vi "Shooter Code.vi"(10 "velocity_lower":dbl=1.0 format="%#_13g", 11 "velocity_upper":dbl=0.9 format="%#_13g") -> (1 "lowerRPM":dbl, 3 "upperRPM":dbl)   [LabVIEW 2015]
panel:
  in  "index":dbl=1.0
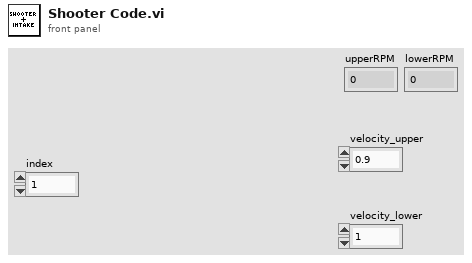
[diagram p1: front panel]
types:
  T1 = typedef "WPI_MotorControlDeviceRef.ctl" = cluster{"DeviceStatus":errorcluster, "Type":T2, "PWM":cluster{"PWM Channel":T3, "DeadBand":T4}, "CAN":cluster{"Device Number":u8, "Control Mode":T5, "Semaphore":T6, "Max Vout":dbl, "TalonSRX Control Mode":T7}, "Invert":bool}
  T2 = typedef "WPI_MotorControlType.ctl" = enum16{"PWM", "CAN", "CANTalonSRX"}
  T3 = typedef "FPGA_DIOPWMChannel.ctl" = enum8{"PWM 0", "PWM 1", "PWM 2", "PWM 3", "PWM 4", "PWM 5", "PWM 6", "PWM 7", "PWM 8", "PWM 9", "PWM MXP 0", "PWM MXP 1", "PWM MXP 2", "PWM MXP 3", "PWM MXP 4", "PWM MXP 5", "PWM MXP 6", "PWM MXP 7", "PWM MXP 8", "PWM MXP 9", "Invalid"}
  T4 = typedef "WPI_PWMDeadband.ctl" = cluster{"Name":string, "maxPositivePwm":i32, "minPositivePwm":i32, "centerPwm":i32, "maxNegativePwm":i32, "minNegativePwm":i32, "angularRange":u16}
  T5 = typedef "WPI_CANJaguar_ControlMode.ctl" = enum8{"Percent VBus", "Current", "Speed", "Position", "Voltage"}
  T6 = typedef "Semaphore RefNum" = refnum<k1>
  T7 = typedef "WPI_CANTalonSRX_APIControlMode.ctl" = enum8{"Percent VBus", "Speed", "Position", "Slave", "Unchanged / Invalid", "Voltage Compensation", "Current", "Motion Profile"}
  T8 = typedef "WPI_CANTalonSRX_GlobalStatus.ctl" = cluster{"Applied Throttle":dbl, "Module Enabled":bool, "CAN Error":errorcluster, "Closed Loop Error":dbl, "Forward Limit Switch Closed":bool, "Reverse Limit Switch Closed":bool, "Sensor Position":dbl, "Sensor Velocity":dbl, "Current":dbl, "Sticky Fault - Over Temp":bool, "Sticky Fault - Under Voltage":bool, "Sticky Fault - Forward Limit":bool, "Sticky Fault - Reverse Limit":bool, "Sticky Fault - Forward Soft Limit":bool, "Sticky Fault - Reverse Soft Limit":bool, "Brake is Enabled":bool, "Encoder Position":dbl, "Encoder Velocity":dbl, "Encoder Index Count":dbl, "Encoder A Pin State":bool, "Encoder B Pin State":bool, "Encoder Index Pin State":bool, "Analog In":dbl, "Analog In Velocity":dbl, "Temperature (C)":dbl, "Battery Voltage":dbl, "Control 5 Is Supported":bool, "Current Profile Slot Select":dbl, "Pos Div 8":bool, "Vel Div 4":bool, "Pulse Width Position":i32, "Pulse Width Velocity":i32, "Pulse Width Rise To Rise (us)":i32, "Pulse Width Rise To Fall (us)":i32, "Mot Prof Active Is Under Run":bool, "Mot Prof Active Has Under Run":bool, "Mot Prof Active Is Last":bool, "Mot Prof Active Velocity Only":bool, "Mot Prof Active Is Valid":bool, "Mot Prof Buffer Is Full":bool, "Mot Prof Active Profile Slot Select":i32, "Mot Prof NextID":i32, "Mot Prof Count":i32, "Mot Prof Active Velocity":dbl, "Mot Prof Active Position":dbl, "Mot Prof Output Enable":i32}
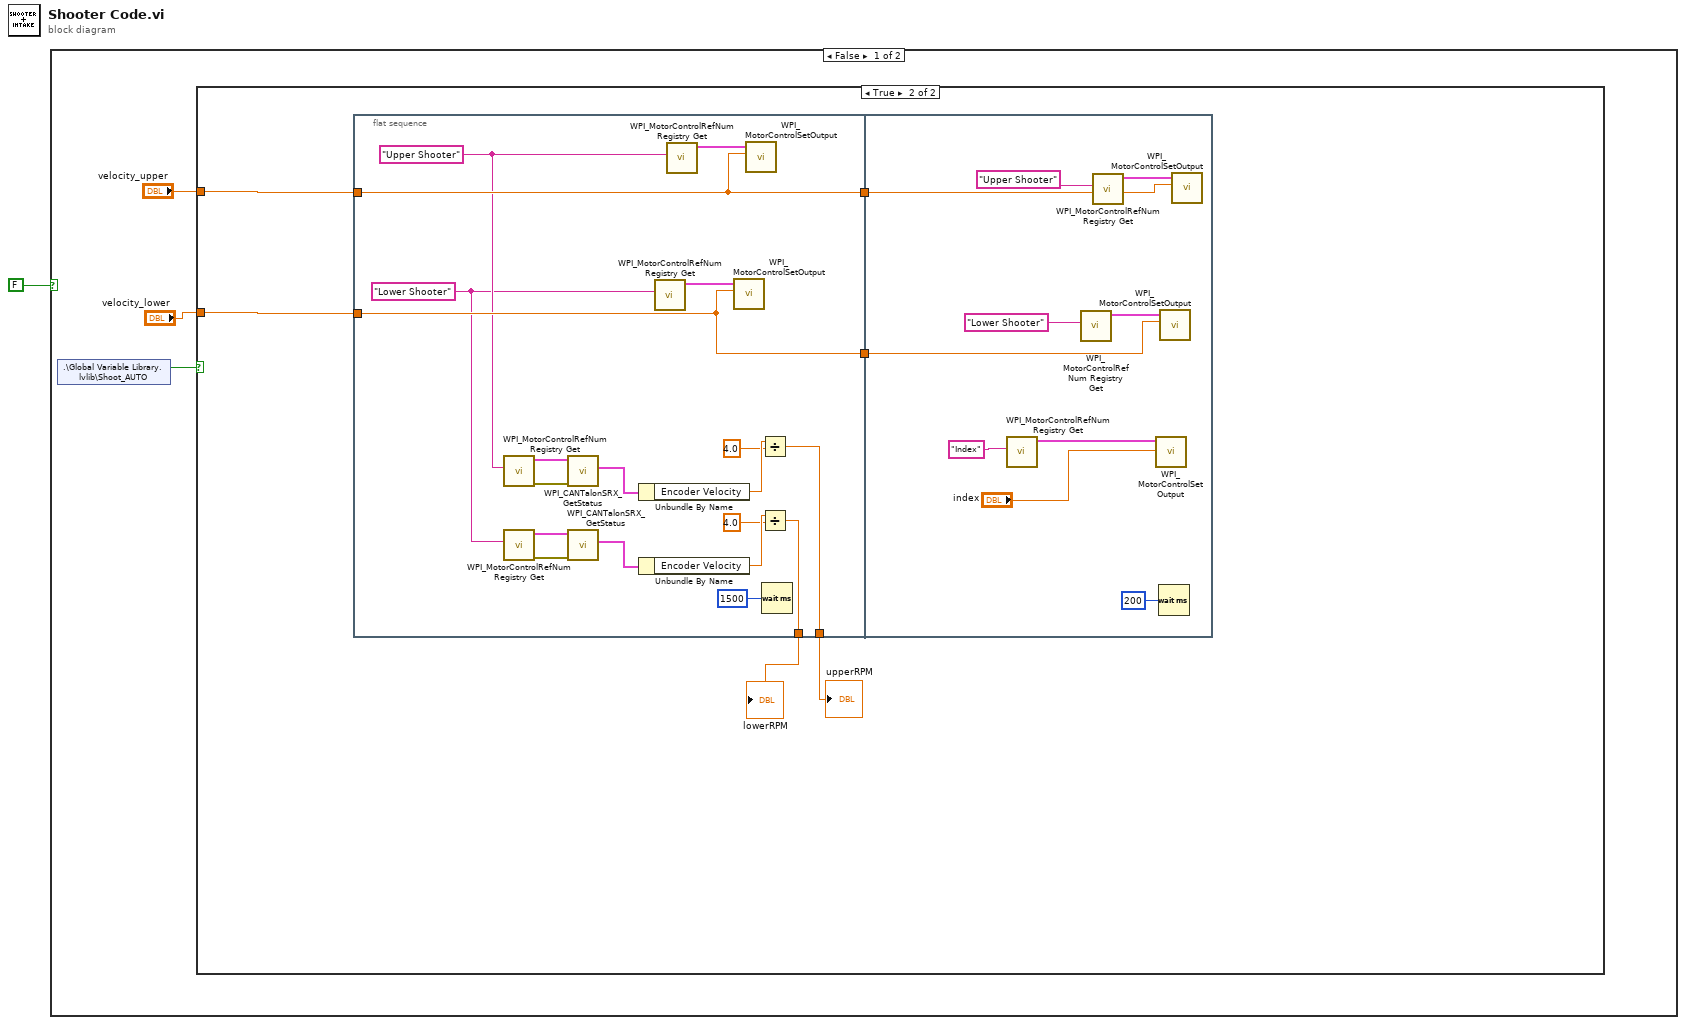
[diagram p0: block diagram]
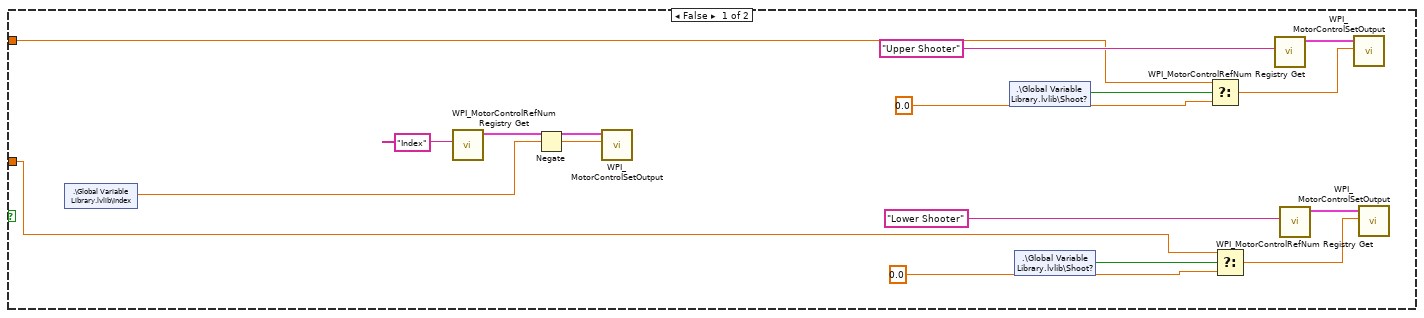
[diagram p2: hidden frame]
diagram:
  n1 = case shown="False" FALSE {
    frame False {
      n2 = shared-variable ".\\Global Variable Library.lvlib\\Shoot_AUTO"() -> (w4:bool)  [unwired: 1 in, 1 out]
      n3 = case shown="True" w4 {
        tunnel: "velocity_lower" -> [w5 w26]
        tunnel: "velocity_upper" -> [w6 w25]
        frame False {
          n4 = shared-variable ".\\Global Variable Library.lvlib\\Index"() -> (w7:dbl)  [unwired: 1 in, 1 out]
          n5 = call <vilib>:"WPI_MotorControlRefNum Registry Get.vi"("refnum name"="Index") -> ("MotorControlDevRef"=w10:T1)  [unwired: 9 in, 1 out]
          n6 = Negate(x=w7) -> (-x=w8:dbl)
          n7 = call <vilib>:"WPI_MotorControlSetOutput.vi"("Output"=w8, "MotorControlDevRef"=w10) -> ()  [unwired: 7 in, 3 out]
          n8 = shared-variable ".\\Global Variable Library.lvlib\\Shoot?"() -> (w18:bool)  [unwired: 1 in, 1 out]
          n9 = shared-variable ".\\Global Variable Library.lvlib\\Shoot?"() -> (w13:bool)  [unwired: 1 in, 1 out]
          n10 = Select(t=w6, s=w18, f=0.0) -> (s? t:f=w20:dbl)
          n11 = Select(t=w5, s=w13, f=0.0 ("f 2")) -> (s? t:f=w11:dbl)
          n12 = call <vilib>:"WPI_MotorControlRefNum Registry Get.vi"("refnum name"="Upper Shooter") -> ("MotorControlDevRef"=w16:T1)  [unwired: 9 in, 1 out]
          n13 = call <vilib>:"WPI_MotorControlRefNum Registry Get.vi"("refnum name"="Lower Shooter") -> ("MotorControlDevRef"=w15:T1)  [unwired: 9 in, 1 out]
          n14 = call <vilib>:"WPI_MotorControlSetOutput.vi"("Output"=w20, "MotorControlDevRef"=w16) -> ()  [unwired: 7 in, 3 out]
          n15 = call <vilib>:"WPI_MotorControlSetOutput.vi"("Output"=w11, "MotorControlDevRef"=w15) -> ()  [unwired: 7 in, 3 out]
        }
        frame True {
          n16 = flat-sequence {
            tunnel: [w43] -> w24
            tunnel: [w42] -> w23
            tunnel: w25 -> [w43]
            tunnel: w26 -> [w42]
            tunnel: [w28] -> w22
            tunnel: [w27] -> w21
            tunnel: w24 -> [w51]
            tunnel: w23 -> [w50]
            frame #0 {
              w35 = "Upper Shooter" ("refnum name")
              w29 = "Lower Shooter" ("refnum name")
              n17 = call <vilib>:"WPI_MotorControlRefNum Registry Get.vi"("refnum name"=w35) -> ("error out"=w38:errorcluster, "MotorControlDevRef"=w39:T1)  [unwired: 9 in]
              n18 = call <vilib>:"WPI_MotorControlRefNum Registry Get.vi"("refnum name"=w29) -> ("error out"=w32:errorcluster, "MotorControlDevRef"=w33:T1)  [unwired: 9 in]
              n19 = call <vilib>:"WPI_CANTalonSRX_GetStatus.vi"("error in (no error)"=w38, "CAN Talon SRX Ref"=w39) -> ("Talon SRX Status"=w40:T8)  [unwired: 7 in, 2 out]
              n20 = call <vilib>:"WPI_CANTalonSRX_GetStatus.vi"("error in (no error)"=w32, "CAN Talon SRX Ref"=w33) -> ("Talon SRX Status"=w34:T8)  [unwired: 7 in, 2 out]
              n21 = Unbundle By Name(w40) -> ("Encoder Velocity"=w37:dbl)
              n22 = Unbundle By Name(w34) -> ("Encoder Velocity"=w31:dbl)
              n23 = call <vilib>:"WPI_MotorControlRefNum Registry Get.vi"("refnum name"=w29) -> ("MotorControlDevRef"=w45:T1)  [unwired: 9 in, 1 out]
              n24 = call <vilib>:"WPI_MotorControlRefNum Registry Get.vi"("refnum name"=w35) -> ("MotorControlDevRef"=w44:T1)  [unwired: 9 in, 1 out]
              n25 = call <vilib>:"WPI_MotorControlSetOutput.vi"("Output"=w42, "MotorControlDevRef"=w45) -> ()  [unwired: 7 in, 3 out]
              n26 = call <vilib>:"WPI_MotorControlSetOutput.vi"("Output"=w43, "MotorControlDevRef"=w44) -> ()  [unwired: 7 in, 3 out]
              n27 = Divide(x=w37, y=4.0) -> (x/y=w27:dbl)
              n28 = Divide(x=w31, y=4.0) -> (x/y=w28:dbl)
              n29 = Wait (ms)(milliseconds to wait=u32 1500) -> ()  [unwired: 1 out]
            }
            frame #1 {
              n30 = call <vilib>:"WPI_MotorControlRefNum Registry Get.vi"("refnum name"="Index") -> ("MotorControlDevRef"=w48:T1)  [unwired: 9 in, 1 out]
              n31 = call <vilib>:"WPI_MotorControlRefNum Registry Get.vi"("refnum name"="Lower Shooter") -> ("MotorControlDevRef"=w53:T1)  [unwired: 9 in, 1 out]
              n32 = call <vilib>:"WPI_MotorControlRefNum Registry Get.vi"("refnum name"="Upper Shooter") -> ("MotorControlDevRef"=w54:T1)  [unwired: 9 in, 1 out]
              n33 = call <vilib>:"WPI_MotorControlSetOutput.vi"("Output"="index", "MotorControlDevRef"=w48) -> ()  [unwired: 7 in, 3 out]
              n34 = Wait (ms)(milliseconds to wait=u32 200) -> ()  [unwired: 1 out]
              n35 = call <vilib>:"WPI_MotorControlSetOutput.vi"("Output"=w50, "MotorControlDevRef"=w53) -> ()  [unwired: 7 in, 3 out]
              n36 = call <vilib>:"WPI_MotorControlSetOutput.vi"("Output"=w51, "MotorControlDevRef"=w54) -> ()  [unwired: 7 in, 3 out]
            }
          }
          "lowerRPM" <- w22
          "upperRPM" <- w21
        }
      }
    }
    frame True {
    }
  }
